vi "WSVCAP SHL Host LL RFFE Read.vi"(0 "RFFE Data [DUT Ordered]":u8[][](array[numeric]) format="%02x", 1 "Wait Ticks":u32, 2 "Slave Address":u8, 5 "Bytes to Read":u8, 7 "Socket Mask [U16]":u16=1 format="%02x", 11 "error in":errorcluster) -> (4 "RFFE Read Data [DUT Ordered]":u8[][](array[numeric]), 8 "Status":u8[](array[numeric]), 15 "error out":errorcluster)   [LabVIEW 2012]
uses:
  Type Defs/WSVCAP SHL Top Level Write Read State Enum.ctl
  Type Defs/WSVCAP SHL State.ctl
  Type Defs/WSVCAP SHL Top Level Control Enum.ctl
  Type Defs/WSVCAP SHL Transaction Enum.ctl
panel:
  out "Write Data":u64[](array[numeric]) format="%032b"
  out "Bit Array":u64[](array[numeric]) format="%.0x"
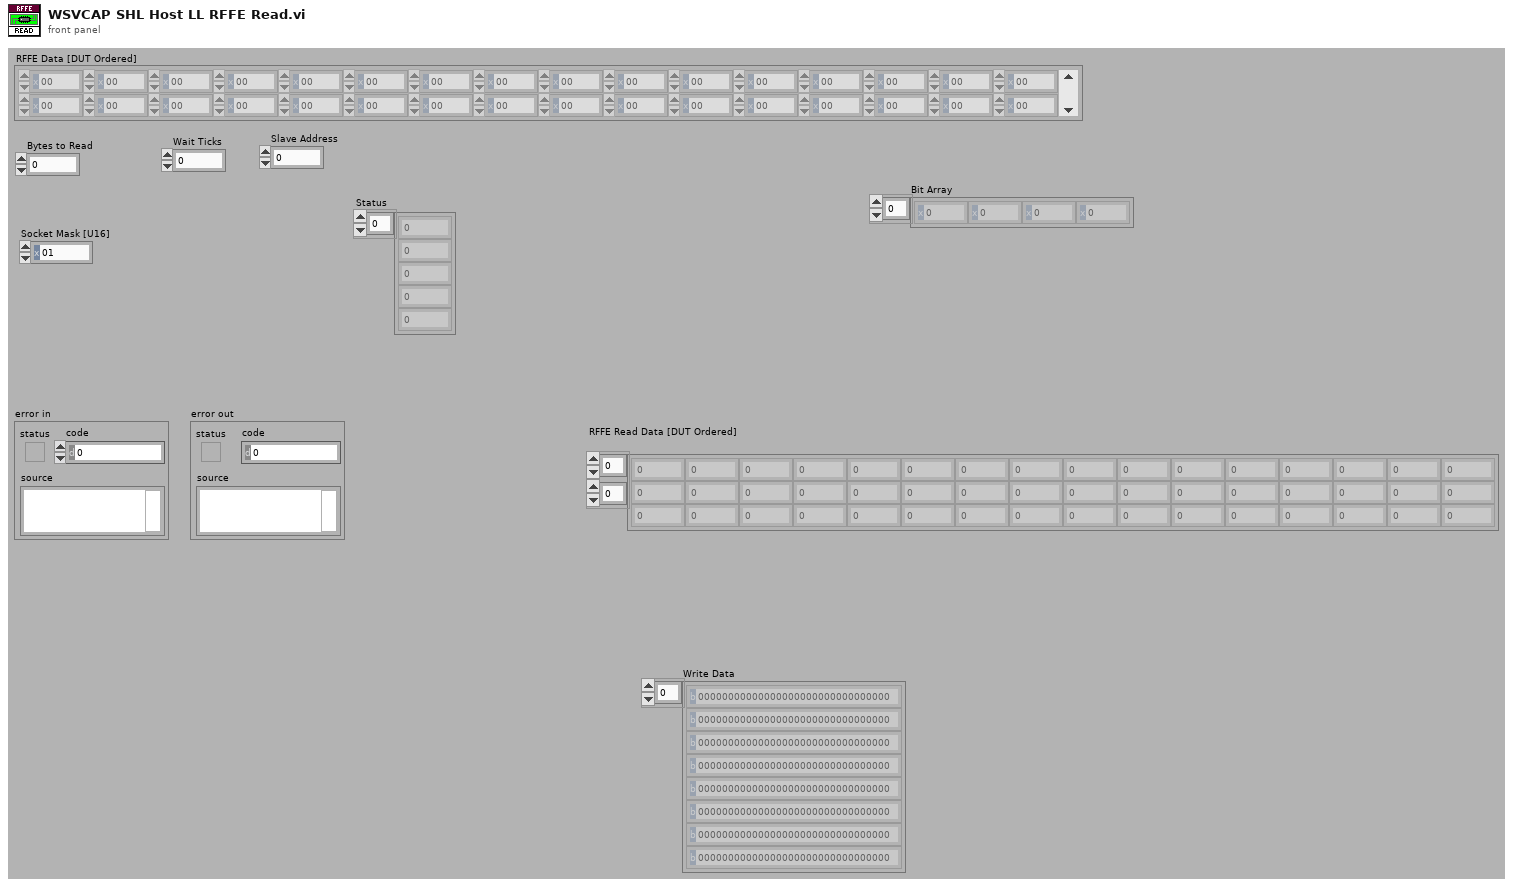
[diagram p1: front panel]
types:
  T1 = typedef "WSVCAP SHL Top Level Write Read State Enum.ctl" = enum16{"Start", "Write", "Read", "Get Status", "Wait Until Done"}
  T2 = typedef "WSVCAP SHL State.ctl" = enum8{"Idle", "Transfer Data"}
  T3 = typedef "WSVCAP SHL Transaction Enum.ctl" = enum16{"I2C-Read Data", "I2C-Write Data", "SPI-Write/Read Data", "RFFE-Ext Write", "RFFE-Ext Read"}
  T4 = typedef "WSVCAP SHL Top Level Control Enum.ctl" = enum16{"Start", "Cmd", "Transaction", "Wait Ticks", "Socket Mask", "Slave Address", "Sub Address", "Bytes to Write", "Bytes to Read", "Write Data", "Write Flag", "Read Data", "Read Flag", "Ack Read", "Read Status Flag", "Ack Read Status", "Status", "Cycle Count", "Stop Cycle", "Exit"}
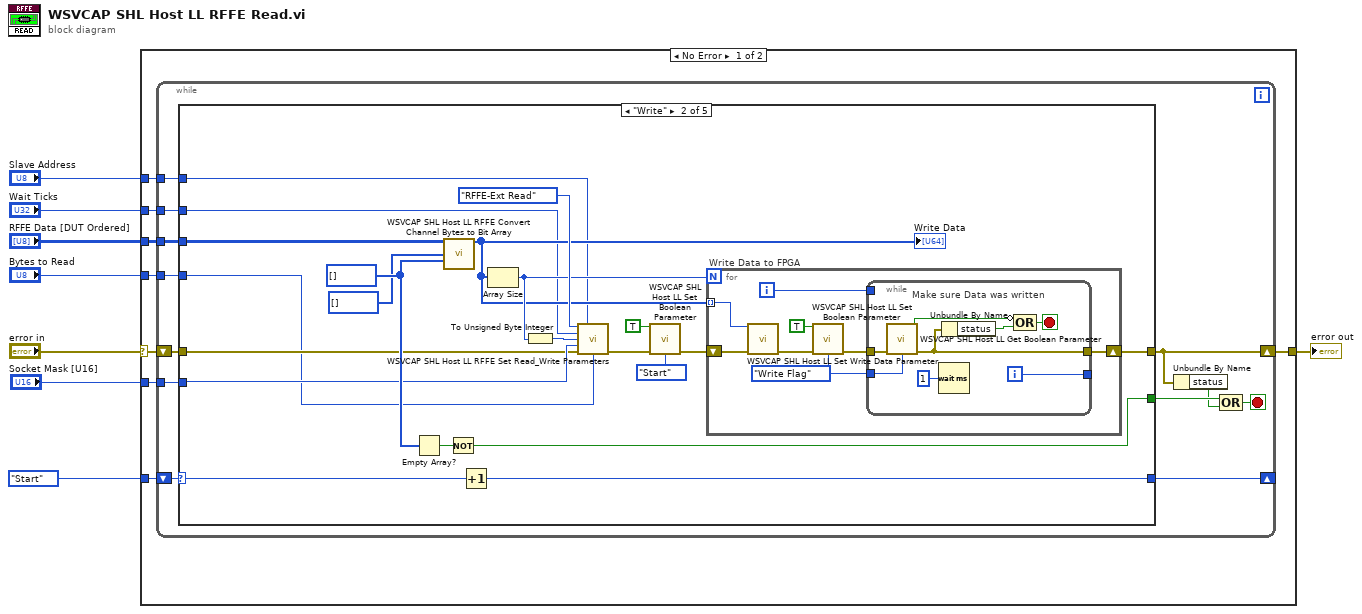
[diagram p0: block diagram]
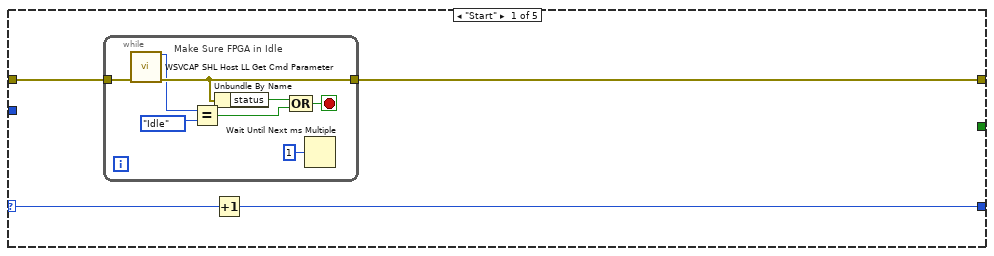
[diagram p2: hidden frame]
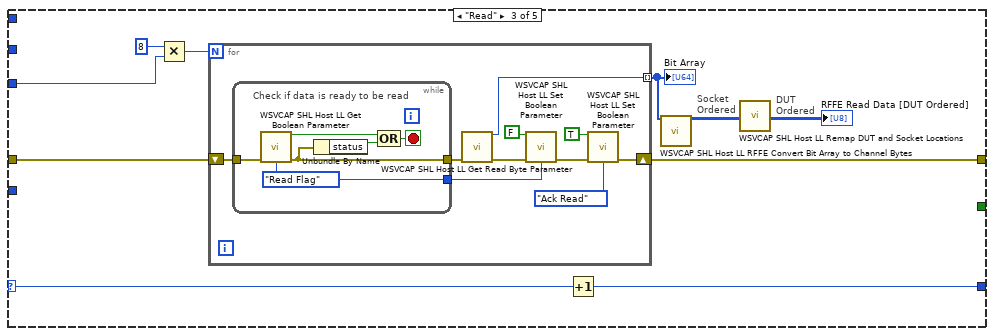
[diagram p3: hidden frame]
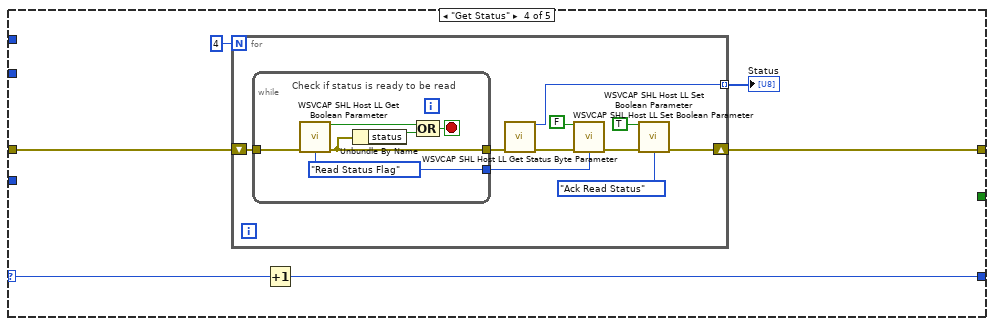
[diagram p4: hidden frame]
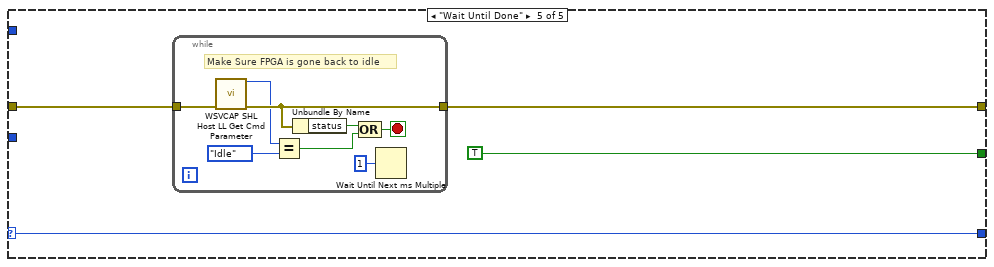
[diagram p5: hidden frame]
diagram:
  n1 = case shown="No Error" "error in" {
    selector: "error in" -> [w13 w138]
    tunnel: [w16 w138] -> w8
    tunnel: WSVCAP_SHL_Top_Level_Write_Read_State_Enum."Start" ("Write Read State") -> [w15 _]
    tunnel: "Socket Mask [U16]" -> [w14 _]
    tunnel: "Wait Ticks" -> [w12 _]
    tunnel: "Bytes to Read" -> [w11 _]
    tunnel: "Slave Address" -> [w10 _]
    tunnel: "RFFE Data [DUT Ordered]" -> [w9 _]
    frame No Error {
      n2 = while {
        shift-right: [w27] -> w16
        shift-left: w13 -> [w28]
        shift-right: [w22] -> _
        shift-left: w15 -> [w23]
        tunnel: w14 -> [w21]
        tunnel: w12 -> [w20]
        tunnel: w11 -> [w19]
        tunnel: w10 -> [w18]
        tunnel: w9 -> [w17]
        stop <- w24 stop-if-true
        n3 = case shown="\"Write\"" w23 {
          selector: w23 -> [w31 w51 w87 w107 w127]
          tunnel: w28 -> [w32 w45 w79 w109 w129]
          tunnel: [w29 w49 w82 w108 w128] -> w27
          tunnel: [_ w42 _ _ TRUE] -> w26
          tunnel: [w30 w43 w86 w106 w127] -> w22
          tunnel: w21 -> [_ w50 _ _ _]
          tunnel: w20 -> [_ w46 _ _ _]
          tunnel: w19 -> [_ w41 w78 _ _]
          tunnel: w18 -> [_ w47 _ _ _]
          tunnel: w17 -> [_ w44 _ _ _]
          frame "Start" {
            n4 = while {
              tunnel: w32 -> [w36]
              tunnel: [w35] -> w29
              stop <- w40 stop-if-true
              # "Make Sure FPGA in Idle"
              n5 = call "WSVCAP SHL Host LL Get Cmd Parameter.vi"("error in (no error)"=w36) -> ("I2C_Cmd"=w34:T2, "error out"=w35:errorcluster)  [unwired: 13 in]
              n6 = Equal?(x=w34, y=WSVCAP_SHL_State."Idle" ("Type")) -> (x = y?=w38:bool)
              n7 = Unbundle By Name(w35) -> ("status"=w33:bool)
              n8 = Compound Arithmetic op=OR(w33, w38) -> (w40:bool)
              n9 = Wait Until Next ms Multiple(millisecond multiple=u32 1) -> ()  [unwired: 1 out]
            }
            n10 = Increment(x=w31) -> (x+1=w30:T1)
          }
          frame "Write" {
            w53 = u32[] [] ("Cycle CMD Delay Out (ticks)")
            # "Write Data to FPGA"
            n11 = Empty Array?(array=w53) -> (empty?=w54:bool)
            n12 = call "WSVCAP SHL Host LL RFFE Convert Channel Bytes to Bit Array.vi"("RFFE Data [DUT Ordered]"=w44, "Cycle CMD Lengths Out (bits)"=u8[] [], "Cycle CMD Delay Out (ticks)"=w53) -> ("Write Data"=w52:u64[])  [unwired: 12 in]
            "Write Data" <- w52
            n13 = Not(x=w54) -> (.not. x?=w42:bool)
            n14 = Increment(x=w51) -> (x+1=w43:T1)
            n15 = Array Size(array=w52) -> (size(s)=w60:i32)
            n16 = To Unsigned Byte Integer(number=w60) -> (unsigned 8bit integer=w58:u8)
            n17 = call "WSVCAP SHL Host LL RFFE Set Read_Write Parameters.vi"("Transaction"=WSVCAP_SHL_Transaction_Enum."RFFE-Ext Read", "Slave Address"=w47, "Wait Ticks"=w46, "Bytes to Write"=w58, "Socket Mask [U16]"=w50, "error in (no error)"=w45, "Bytes to Read (Ext-Read Only)"=w41) -> ("error out"=w55:errorcluster)  [unwired: 8 in]
            n18 = call "WSVCAP SHL Host LL Set Boolean Parameter.vi"("Boolean In"=TRUE, "error in (no error)"=w55, "FPGA Top Level Control"=WSVCAP_SHL_Top_Level_Control_Enum."Start") -> ("error out"=w59:errorcluster)  [unwired: 12 in]
            n19 = for {
              N: w60 -> [_]
              shift-right: [w69] -> w49
              shift-left: w59 -> [w68]
              tunnel: w52 -> [w67] mode=indexing
              i -> [w62]
              w63 = WSVCAP_SHL_Top_Level_Control_Enum."Write Flag" ("FPGA Top Level Control")
              n20 = call "WSVCAP SHL Host LL Set Write Data Parameter.vi"("Write Byte In"=w67, "error in (no error)"=w68) -> ("error out"=w66:errorcluster)  [unwired: 13 in]
              n21 = call "WSVCAP SHL Host LL Set Boolean Parameter.vi"("Boolean In"=TRUE, "error in (no error)"=w66, "FPGA Top Level Control"=w63) -> ("error out"=w64:errorcluster)  [unwired: 12 in]
              n22 = while {
                tunnel: w64 -> [w75]
                tunnel: [w74] -> w69
                tunnel: w63 -> [w72]
                tunnel: w62 -> [_]
                tunnel: [w70] -> _
                i -> [w70]
                stop <- w77 stop-if-true
                # "Make sure Data was written"
                n23 = call "WSVCAP SHL Host LL Get Boolean Parameter.vi"("error in (no error)"=w75, "FPGA Top Level Control"=w72) -> ("Boolean Out"=w73:bool, "error out"=w74:errorcluster)  [unwired: 12 in]
                n24 = Wait (ms)(milliseconds to wait=u32 1) -> ()  [unwired: 1 out]
                n25 = Unbundle By Name(w74) -> ("status"=w71:bool)
                n26 = Compound Arithmetic op=OR(invert w73, w71) -> (w77:bool)
              }
            }
          }
          frame "Read" {
            # "DUT\nOrdered"
            # "Socket\nOrdered"
            n27 = Multiply(x=8, y=w78) -> (x*y=w84:i32)
            n28 = for {
              N: w84 -> [_]
              shift-right: [w94] -> w82
              shift-left: w79 -> [w97]
              tunnel: [w88] -> w85 mode=indexing
              n29 = while {
                tunnel: w97 -> [w101]
                tunnel: [w100] -> w96
                tunnel: [w98] -> w93
                stop <- w103 stop-if-true
                w98 = WSVCAP_SHL_Top_Level_Control_Enum."Read Flag" ("FPGA Top Level Control")
                # "Check if data is ready to be read"
                n30 = call "WSVCAP SHL Host LL Get Boolean Parameter.vi"("error in (no error)"=w101, "FPGA Top Level Control"=w98) -> ("Boolean Out"=w102:bool, "error out"=w100:errorcluster)  [unwired: 12 in]
                n31 = Unbundle By Name(w100) -> ("status"=w99:bool)
                n32 = Compound Arithmetic op=OR(w102, w99) -> (w103:bool)
              }
              n33 = call "WSVCAP SHL Host LL Get Read Byte Parameter.vi"("error in (no error)"=w96) -> ("Read Data In"=w88:u64, "error out"=w95:errorcluster)  [unwired: 13 in]
              n34 = call "WSVCAP SHL Host LL Set Boolean Parameter.vi"("Boolean In"=FALSE ("Read Flag"), "error in (no error)"=w95, "FPGA Top Level Control"=w93) -> ("error out"=w89:errorcluster)  [unwired: 12 in]
              n35 = call "WSVCAP SHL Host LL Set Boolean Parameter.vi"("Boolean In"=TRUE ("Write Flag"), "error in (no error)"=w89, "FPGA Top Level Control"=WSVCAP_SHL_Top_Level_Control_Enum."Ack Read") -> ("error out"=w94:errorcluster)  [unwired: 12 in]
            }
            "Bit Array" <- w85
            n36 = Increment(x=w87) -> (x+1=w86:T1)
            n37 = call "WSVCAP SHL Host LL RFFE Convert Bit Array to Channel Bytes.vi"("Bit Array"=w85) -> ("RFFE Read Data [Socket Ordered]"=w81:u8[][])  [unwired: 14 in]
            n38 = call "WSVCAP SHL Host LL Remap DUT and Socket Locations.vi"("C1 Socket Ordered Data In"=w81) -> ("C1 DUT Ordered Data Out"=→"RFFE Read Data [DUT Ordered]":u8[][])  [unwired: 13 in, 5 out]
          }
          frame "Get Status" {
            n39 = for {
              N: 4 -> [_]
              shift-right: [w118] -> w108
              shift-left: w109 -> [w119]
              tunnel: [w110] -> w104 mode=indexing
              n40 = while {
                tunnel: w119 -> [w123]
                tunnel: [w122] -> w117
                tunnel: [w120] -> w115
                stop <- w125 stop-if-true
                w120 = WSVCAP_SHL_Top_Level_Control_Enum."Read Status Flag" ("FPGA Top Level Control")
                # "Check if status is ready to be read"
                n41 = call "WSVCAP SHL Host LL Get Boolean Parameter.vi"("error in (no error)"=w123, "FPGA Top Level Control"=w120) -> ("Boolean Out"=w124:bool, "error out"=w122:errorcluster)  [unwired: 12 in]
                n42 = Unbundle By Name(w122) -> ("status"=w121:bool)
                n43 = Compound Arithmetic op=OR(w124, w121) -> (w125:bool)
              }
              n44 = call "WSVCAP SHL Host LL Get Status Byte Parameter.vi"("error in (no error)"=w117) -> ("I2C Status Byte"=w110:u8, "error out"=w116:errorcluster)  [unwired: 13 in]
              n45 = call "WSVCAP SHL Host LL Set Boolean Parameter.vi"("Boolean In"=FALSE ("Read Flag"), "error in (no error)"=w116, "FPGA Top Level Control"=w115) -> ("error out"=w111:errorcluster)  [unwired: 12 in]
              n46 = call "WSVCAP SHL Host LL Set Boolean Parameter.vi"("Boolean In"=TRUE ("Write Flag"), "error in (no error)"=w111, "FPGA Top Level Control"=WSVCAP_SHL_Top_Level_Control_Enum."Ack Read Status") -> ("error out"=w118:errorcluster)  [unwired: 12 in]
            }
            "Status" <- w104
            n47 = Increment(x=w107) -> (x+1=w106:T1)
          }
          frame "Wait Until Done" {
            n48 = while {
              tunnel: w129 -> [w132]
              tunnel: [w131] -> w128
              stop <- w134 stop-if-true
              # "Make Sure FPGA is gone back to idle"
              n49 = call "WSVCAP SHL Host LL Get Cmd Parameter.vi"("error in (no error)"=w132) -> ("I2C_Cmd"=w130:T2, "error out"=w131:errorcluster)  [unwired: 13 in]
              n50 = Equal?(x=w130, y=WSVCAP_SHL_State."Idle") -> (x = y?=w135:bool)
              n51 = Unbundle By Name(w131) -> ("status"=w136:bool)
              n52 = Compound Arithmetic op=OR(w136, w135) -> (w134:bool)
              n53 = Wait Until Next ms Multiple(millisecond multiple=u32 1) -> ()  [unwired: 1 out]
            }
          }
        }
        n54 = Unbundle By Name(w27) -> ("status"=w25:bool)
        n55 = Compound Arithmetic op=OR(w26, w25) -> (w24:bool)
      }
    }
    frame Error {
    }
  }
  "error out" <- w8
